vi "DTS_Test.vi"(10 "PEU":refnum<class "PEU.lvclass">, 11 "E5071C":refnum<class "E5071C.lvclass">) -> ()   [LabVIEW 2020]
uses:
  Driver/E5071C/E5071C/E5071C.lvclass
  Driver/PEU/PEU/PEU.lvclass
panel:
  in  "Title":string="开关自动测试"
  in  "负载选择":enum32{"No Selection", "Item 0", "Item 1"}(radio)=enum."Item 0"
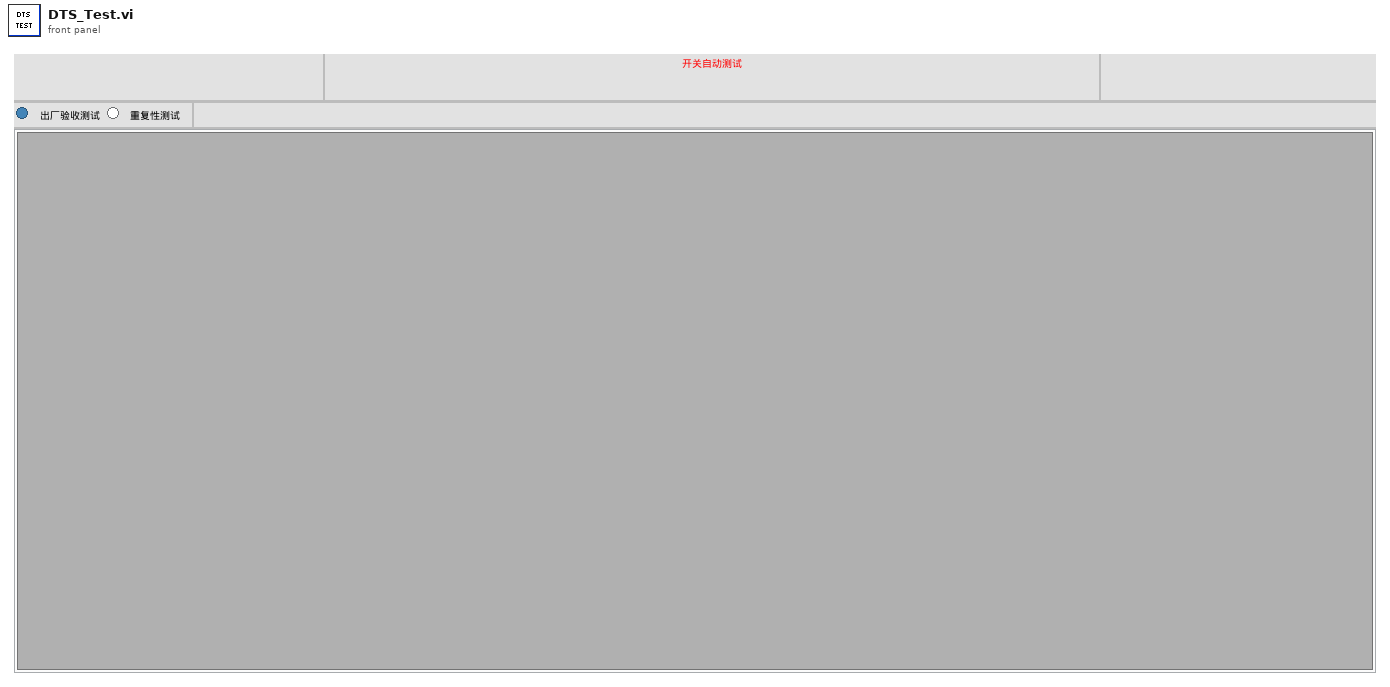
[diagram p1: front panel]
types:
  T1 = cluster{"E5071C":refnum<class "E5071C.lvclass">, "TP":string, "TPs":string[], "PEU":refnum<class "PEU.lvclass">}
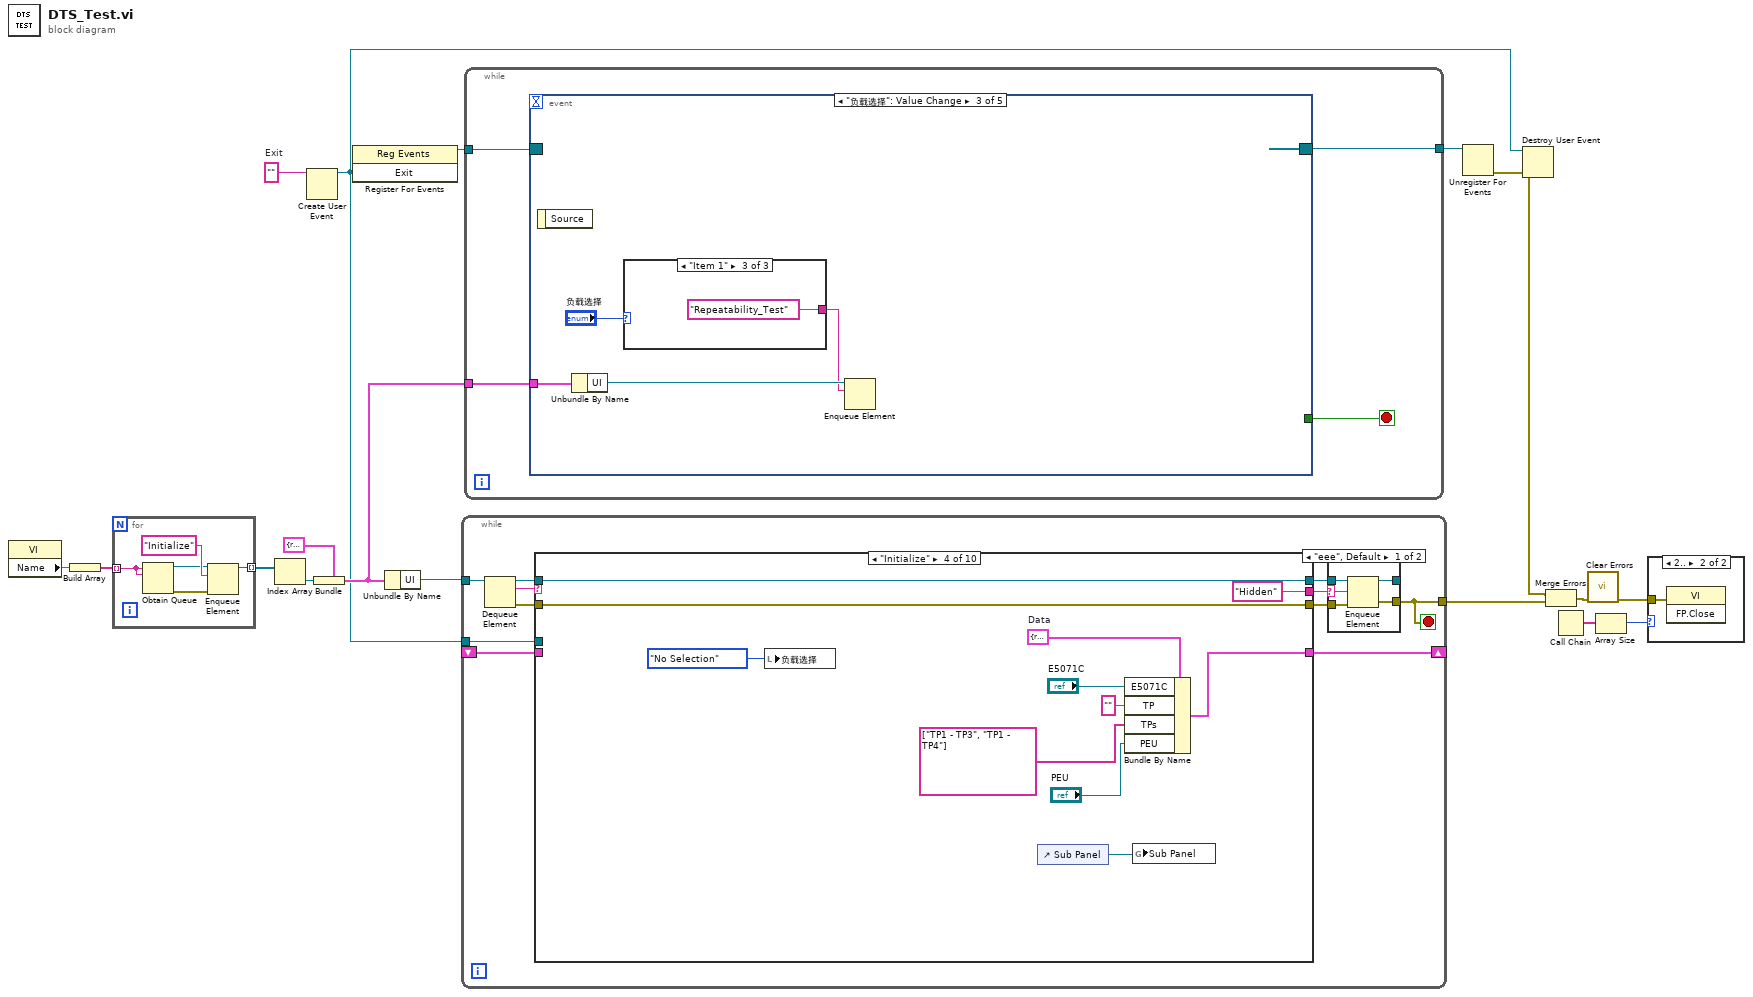
[diagram p0: block diagram]
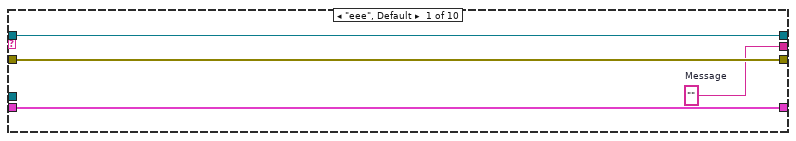
[diagram p4: hidden frame]
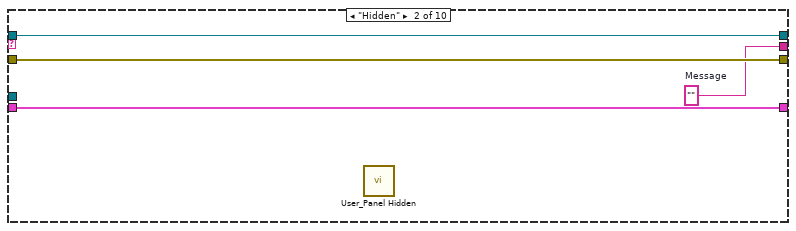
[diagram p5: hidden frame]
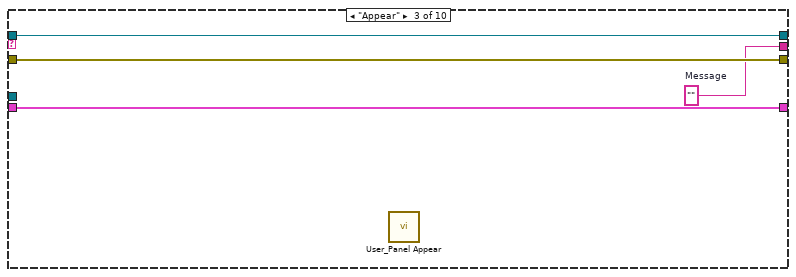
[diagram p6: hidden frame]
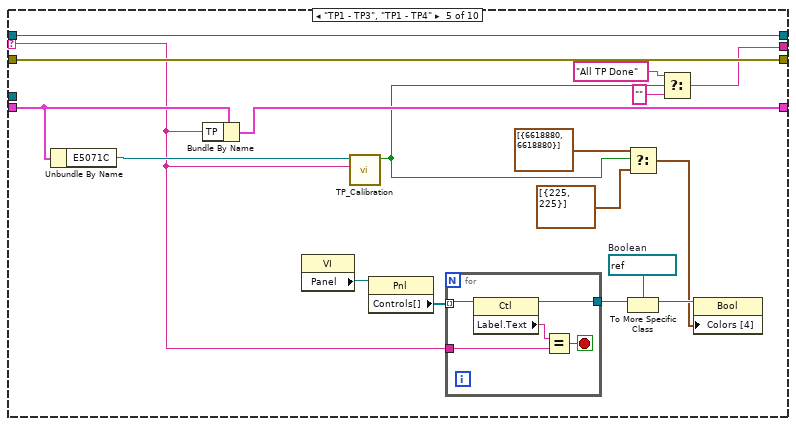
[diagram p7: hidden frame]
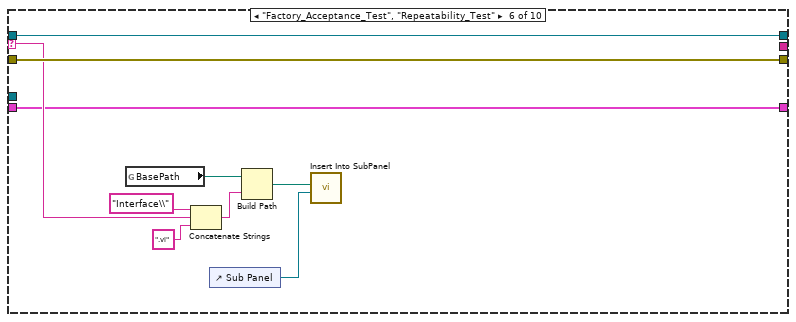
[diagram p8: hidden frame]
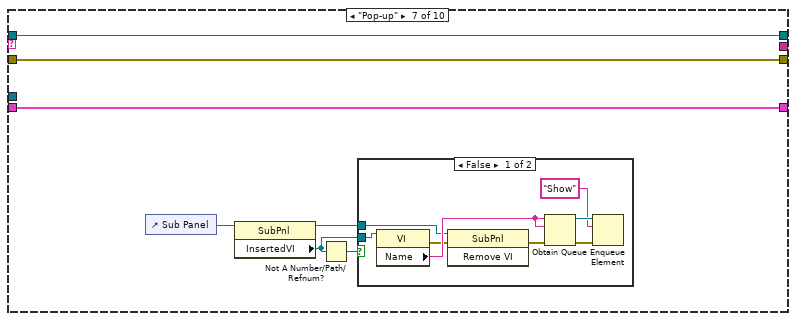
[diagram p9: hidden frame]
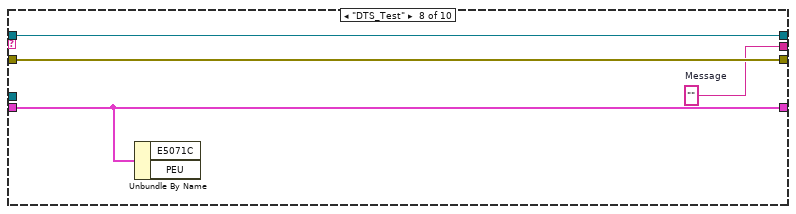
[diagram p11: hidden frame]
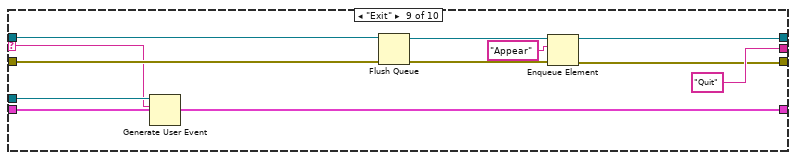
[diagram p12: hidden frame]
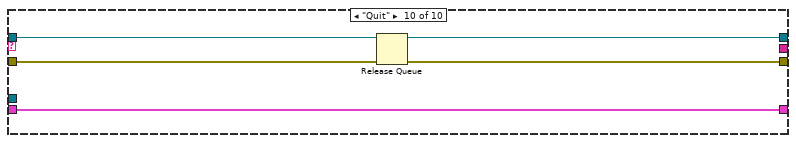
[diagram p13: hidden frame]
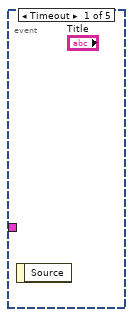
[diagram p14: hidden frame]
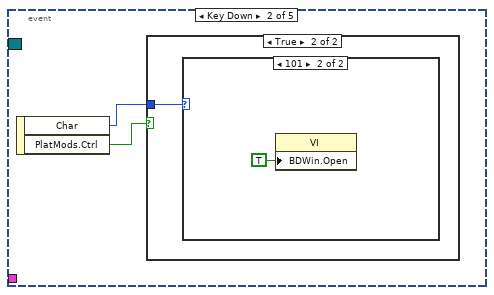
[diagram p15: hidden frame]
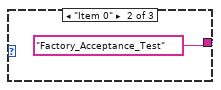
[diagram p19: hidden frame]
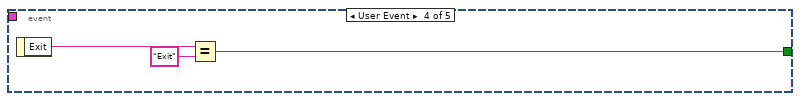
[diagram p20: hidden frame]
diagram:
  w7 = ""  # Exit
  n1 = property class="VI"() -> ("Name"=w17:string)  [unwired: 2 in, 2 out]
  n2 = Build Array(w17) -> (w18:string[])
  n3 = for {
    tunnel: w18 -> [w19] mode=indexing
    tunnel: [w20] -> w12 mode=indexing
    n4 = Obtain Queue(name (unnamed)=w19, element data type=w19) -> (queue out=w22:refnum<queue>, error out=w21:errorcluster)  [unwired: 3 in, 1 out]
    n5 = Enqueue Element(queue=w22, element="Initialize" ("元素"), error in (no error)=w21) -> (queue out=w20:refnum<queue>)  [unwired: 1 in, 2 out]
  }
  n6 = Index Array(array=w12) -> (element=w15:refnum<queue>)  [unwired: 1 in]
  n7 = Create User Event(user event datatype=w7) -> (user event=w11:refnum<user-event>)  [unwired: 1 in, 1 out]
  n8 = Bundle(cluster=cluster{"UI":refnum<queue>} {"UI"=refnum}, "UI"=w15) -> (w16:cluster{"UI":refnum<queue>})
  n9 = register-events(w11) -> (reference out=w8:refnum<event-registration>)  [unwired: 2 in, 1 out]
  n10 = Unbundle By Name(w16) -> ("UI"=w13:refnum<queue>)
  n11 = while {
    tunnel: w13 -> [w34]
    tunnel: [w24] -> w1
    shift-right: [w28] -> _
    shift-left: _ -> [w27]
    tunnel: w11 -> [w26]
    stop <- w24 stop-if-true
    n12 = Dequeue Element(queue=w34) -> (queue out=w33:refnum<queue>, element=w25:string, error out=w30:errorcluster)  [unwired: 2 in, 1 out]
    n13 = case shown="\"Initialize\"" w25 {
      selector: w25 -> [_ _ _ _ w70 w94 _ _ w122 _]
      tunnel: w33 -> [w45 w49 w53 w64 w82 w97 w104 w116 w125 w131]
      tunnel: [w45 w49 w53 w64 w82 w97 w104 w116 w117 w131] -> w32
      tunnel: [w44 w48 w52 w63 w81 w96 w103 w115 w118 w128] -> w31
      tunnel: w30 -> [w44 w48 w52 w63 w81 w96 w103 w115 w124 w130]
      tunnel: [w43 w47 w51 "Hidden" ("Message") w66 _ _ w114 "Quit" ("Message") _] -> w29
      tunnel: [w42 w46 w50 w61 w69 w91 w102 w113 w127 w129] -> w28
      tunnel: w27 -> [w42 w46 w50 _ w71 w91 w102 w113 w127 w129]
      tunnel: w26 -> [_ _ _ _ _ _ _ _ w123 _]
      frame "eee", Default {
        w43 = ""  # Message
      }
      frame "Hidden" {
        w47 = ""  # Message
        n14 = call "User_Panel Hidden.vi"() -> ()  [unwired: 11 in, 1 out]
      }
      frame "Appear" {
        w51 = ""  # Message
        n15 = call "User_Panel Appear.vi"() -> ()  [unwired: 11 in, 1 out]
      }
      frame "Initialize" {
        w62 = T1 {"E5071C"=refnum, "TP"="", "TPs"=["TP1 - TP3", "TP1 - TP4", "TP1 - TP5", "TP1 - TP6", "TP1 - TP7", "TP1 - TP8", "TP1 - TP9", "TP1 - TP10", "TP1 - TP11", "TP1 - TP12", "TP1 - TP13", "TP1 - TP14", "TP2 - TP3", "TP2 - TP4"], "PEU"=refnum}  # Data
        n16 = local write "负载选择"(enum32{"No Selection", "Item 0", "Item 1"}."No Selection" ("负载选择")) -> ()
        n17 = control-ref of="Sub Panel"() -> (w54:refnum<vi>)
        n18 = Bundle By Name(cluster=w62, "E5071C"="E5071C", "TP"="", "TPs"=string[] ["TP1 - TP3", "TP1 - TP4"], "PEU"="PEU") -> (w61:T1)
        n19 = global write "Global.vi" "Sub Panel"(w54) -> ()
      }
      frame "TP1 - TP3", "TP1 - TP4" {
        w77 = refnum<vi> refnum  # Boolean
        n20 = Unbundle By Name(w71) -> ("E5071C"=w80:refnum<class "E5071C.lvclass">)
        n21 = Bundle By Name(cluster=w71, "TP"=w70) -> (w69:T1)
        n22 = property class="VI"() -> ("Panel"=w79:refnum<vi>)  [unwired: 2 in, 2 out]
        n23 = call "TP_Calibration.vi"("TP"=w70, "E5071C"=w80) -> ("Calibration Done"=w68:bool)  [unwired: 9 in]
        n24 = property class="Pnl"(reference=w79) -> ("Controls[]"=w78:refnum<vi>[])  [unwired: 1 in, 2 out]
        n25 = for {
          tunnel: w78 -> [w87] mode=indexing
          tunnel: w70 -> [w85]
          tunnel: [w83] -> w76
          stop <- w84 stop-if-true
          n26 = property class="Ctl"(reference=w87) -> (reference out=w83:refnum<vi>, "Label.Text"=w86:string)  [unwired: 1 in, 1 out]
          n27 = Equal?(x=w86, y=w85) -> (x = y?=w84:bool)
        }
        n28 = Select(t=cluster{u32, u32}[] [{6618880, 6618880}] ("Colors [4]"), s=w68, f=cluster{u32, u32}[] [{225, 225}] ("Colors [4]")) -> (s? t:f=w72:cluster{u32, u32}[])
        n29 = To More Specific Class(target class=w77, reference=w76) -> (specific class reference=w75:refnum<vi>)  [unwired: 1 in, 1 out]
        n30 = Select(t="All TP Done" ("Message"), s=w68, f="") -> (s? t:f=w66:string)
        n31 = property class="Bool"(reference=w75, "Colors [4]"=w72) -> ()  [unwired: 1 in, 2 out]
      }
      frame "Factory_Acceptance_Test", "Repeatability_Test" {
        n32 = global read "Global.vi" "BasePath"() -> (w88:path)
        n33 = Concatenate Strings("Interface\\" ("string"), w94, ".vi" ("string")) -> (w92:string)
        n34 = control-ref of="Sub Panel"() -> (w95:refnum<vi>)
        n35 = Build Path(base path=w88, name or relative path=w92) -> (appended path=w90:path)
        n36 = call "Insert Into SubPanel.vi"("SubPanel Ref"=w95, "VI Path"=w90) -> ()  [unwired: 9 in, 1 out]
      }
      frame "Pop-up" {
        n37 = control-ref of="Sub Panel"() -> (w98:refnum<vi>)
        n38 = property class="SubPnl"(reference=w98) -> (reference out=w101:refnum<vi>, "InsertedVI"=w100:refnum<vi>)  [unwired: 1 in, 1 out]
        n39 = Not A Number/Path/Refnum?(number/path/refnum=w100) -> (NaN/Path/Refnum?=w99:bool)
        n40 = case shown="False" w99 {
          tunnel: w100 -> [w107 _]
          tunnel: w101 -> [w108 _]
          frame False {
            n41 = property class="VI"(reference=w107) -> (error out=w106:errorcluster, "Name"=w110:string)  [unwired: 1 in, 1 out]
            n42 = invoke class="SubPnl" method="Remove VI"(reference=w108, error in=w106) -> (error out=w105:errorcluster)  [unwired: 1 in, 2 out]
            n43 = Obtain Queue(name (unnamed)=w110, element data type=w110, error in (no error)=w105) -> (queue out=w111:refnum<queue>, error out=w112:errorcluster)  [unwired: 2 in, 1 out]
            n44 = Enqueue Element(queue=w111, element="Show" ("元素"), error in (no error)=w112) -> ()  [unwired: 1 in, 3 out]
          }
          frame True {
          }
        }
      }
      frame "DTS_Test" {
        w114 = ""  # Message
        n45 = Unbundle By Name(w113) -> ()  [unwired: 2 out]
      }
      frame "Exit" {
        n46 = Generate User Event(user event=w123, event data cluster=w122) -> ()  [unwired: 2 in, 2 out]
        n47 = Flush Queue(queue=w125, error in (no error)=w124) -> (queue out=w120:refnum<queue>, error out=w119:errorcluster)  [unwired: 1 out]
        n48 = Enqueue Element(queue=w120, element="Appear" ("元素"), error in (no error)=w119) -> (queue out=w117:refnum<queue>, error out=w118:errorcluster)  [unwired: 1 in, 1 out]
      }
      frame "Quit" {
        n49 = Release Queue(queue=w131, error in (no error)=w130) -> (error out=w128:errorcluster)  [unwired: 1 in, 2 out]
      }
    }
    n50 = case shown="\"eee\", Default" w29 {
      selector: w29 -> [w35 _]
      tunnel: w32 -> [w39 w41]
      tunnel: w31 -> [w38 w40]
      tunnel: [w37 w40] -> w24
      tunnel: [w36 w41] -> _
      frame "eee", Default {
        n51 = Enqueue Element(queue=w39, element=w35, error in (no error)=w38) -> (queue out=w36:refnum<queue>, error out=w37:errorcluster)  [unwired: 1 in, 1 out]
      }
      frame "" {
      }
    }
  }
  n52 = while {
    tunnel: w8 -> [w134]
    tunnel: [w133] -> w10
    tunnel: w16 -> [w132]
    stop <- w135 stop-if-true
    n53 = event shown="[2] \"负载选择\": Value Change" {
      selector: w134 -> [_ _ _ _ _]
      dyn-events: [_ _ _ _ _] -> w133
      timeout: _ -> [_ _ _ _ _]
      tunnel: [_ _ _ w147 _] -> w135
      tunnel: w132 -> [_ _ w143 _ w151]
      event Timeout {
        n54 = event-data() -> ()  [unwired: 1 in, 1 out]
      }
      event Key Down {
        n55 = event-data() -> ("Char"=w137:i16, "PlatMods.Ctrl"=w136:bool)  [unwired: 1 in]
        n56 = case shown="True" w136 {
          tunnel: w137 -> [_ w138]
          frame False {
          }
          frame True {
            n57 = case shown="101" w138 {
              frame 0, Default {
              }
              frame 101 {
                n58 = property class="VI"("BDWin.Open"=TRUE ("程序框图窗口:打开")) -> ()  [unwired: 2 in, 2 out]
              }
            }
          }
        }
      }
      event "负载选择": Value Change {
        n59 = event-data() -> ()  [unwired: 1 in, 1 out]
        n60 = Unbundle By Name(w143) -> ("UI"=w141:refnum<queue>)
        n61 = case shown="\"Item 1\"" "负载选择" {
          tunnel: [_ "Factory_Acceptance_Test" ("TP") "Repeatability_Test" ("TP")] -> w140
          frame "No Selection", Default {
          }
          frame "Item 0" {
          }
          frame "Item 1" {
          }
        }
        n62 = Enqueue Element(queue=w141, element=w140) -> ()  [unwired: 2 in, 3 out]
      }
      event User Event {
        n63 = event-data() -> ("Exit"=w148:string)  [unwired: 1 in]
        n64 = Equal?(x=w148, y="Exit") -> (x = y?=w147:bool)
      }
      event Panel Close? {
        n65 = event-data() -> ()  [unwired: 1 in, 1 out]
        n66 = Cluster To Array(cluster=w151) -> (array=w150:refnum<queue>[])
        n67 = for {
          tunnel: w150 -> [w154] mode=indexing
          tunnel: "Exit" ("元素") -> [w153]
          n68 = Enqueue Element(queue=w154, element=w153) -> ()  [unwired: 2 in, 3 out]
        }
        n69 = event-data("Discard?"=TRUE ("放弃？")) -> ()  [unwired: 1 in, 1 out]
      }
    }
  }
  n70 = Unregister For Events(event registration refnum=w10) -> (error out=w9:errorcluster)  [unwired: 1 in]
  n71 = Destroy User Event(user event=w11, error in=w9) -> (error out=w2:errorcluster)
  n72 = Merge Errors(w2, w1) -> (w6:errorcluster)
  n73 = Call Chain() -> (call chain=w4:string[])
  n74 = call <vilib>:"Clear Errors.vi"("error in (no error)"=w6) -> ("error out"=w5:errorcluster)  [unwired: 5 in, 1 out]
  n75 = Array Size(array=w4) -> (size(s)=w3:i32)
  n76 = case shown="2.." w3 {
    tunnel: w5 -> [_ w155]
    frame 0, Default {
    }
    frame 2.. {
      n77 = invoke class="VI" method="FP.Close"(error in=w155) -> ()  [unwired: 2 in, 3 out]
    }
  }
